vi "FGV Actor Classes-Messages.vi"(8 "Error In":errorcluster, 9 "CS++Messages":refnum<class "Message.lvclass">[](array[class]), 10 "Class Name":string, 11 "Action (read)":T1=enum."read") -> (0 "Error Out":errorcluster, 1 "CS++Messages":refnum<class "Message.lvclass">[](array[class]), 2 "Success":bool, 4 "Class Names":string[](array[string]), 6 "CS++Messages":refnum<class "Message.lvclass">[][](array[class]))   [LabVIEW 2016, in "CS++Base.lvlib"]
doc: "This is a FGV to be used to maintain a list of actor classes and corresponding messages."
uses:
  CS++Base.lvlib
  FGV Action.ctl
  <vilib>/ActorFramework/Message/Message.lvclass
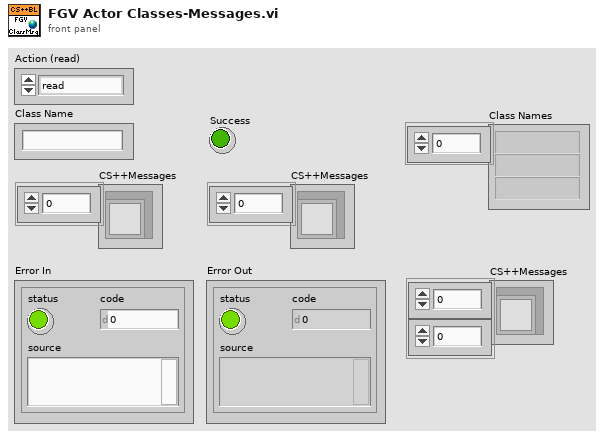
[diagram p1: front panel]
types:
  T1 = typedef "CS++Base.lvlib/FGV Action.ctl" = enum16{"add", "replace", "read", "remove", "reset", "get attributes"}
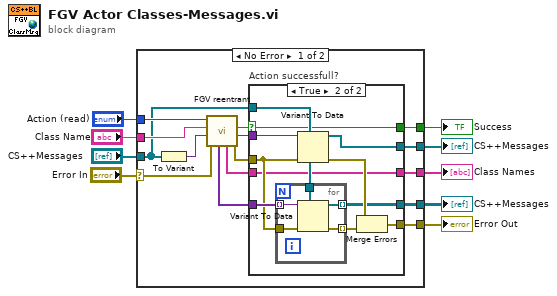
[diagram p0: block diagram]
diagram:
  n1 = case shown="No Error" "Error In" {
    selector: "Error In" -> [w23 w43]
    tunnel: "Action (read)" -> [w24 _]
    tunnel: "Class Name" -> [w22 _]
    tunnel: "CS++Messages" -> [w19 w44]
    tunnel: [w16 w43] -> w5
    tunnel: [w15 _] -> w4
    tunnel: [w14 _] -> w3
    tunnel: [w11 _] -> w2
    tunnel: [w10 w44] -> w1
    frame No Error {
      n2 = To Variant(anything=w19) -> (Variant=w21:variant)
      n3 = call "FGV reentrant.vi"("Error In"=w23, "Data in"=w21, "Attribute Name"=w22, "Action (read)"=w24) -> ("Error Out"=w17:errorcluster, "Data out"=w20:variant, "Success"=w12:bool, "Attribute Names"=w13:string[], "Attribute Values"=w18:variant[])  [unwired: 3 in]
      n4 = case "Action successfull?" shown="True" w12 {
        selector: w12 -> [w26 w28]
        tunnel: w20 -> [_ w37]
        tunnel: w19 -> [_ w36]
        tunnel: w18 -> [_ w35]
        tunnel: w17 -> [w25 w34]
        tunnel: [w25 w31] -> w16
        tunnel: [_ w30] -> w15
        tunnel: [_ w29] -> w14
        tunnel: w13 -> [_ w29]
        tunnel: [w26 w28] -> w11
        tunnel: [_ w27] -> w10
        frame False {
        }
        frame True {
          n5 = for {
            tunnel: w36 -> [w42]
            tunnel: w35 -> [w41] mode=indexing
            tunnel: w34 -> [w40]
            tunnel: [w39] -> w33 mode=indexing
            tunnel: [w38] -> w30 mode=indexing
            n6 = Variant To Data(error in=w40, type=w42, Variant=w41) -> (data=w38:refnum<class "Message.lvclass">[], error out=w39:errorcluster)
          }
          n7 = Variant To Data(error in=w34, type=w36, Variant=w37) -> (data=w27:refnum<class "Message.lvclass">[], error out=w32:errorcluster)
          n8 = Merge Errors(w32, w33) -> (w31:errorcluster)
        }
      }
    }
    frame Error {
    }
  }
  "Error Out" <- w5
  "Class Names" <- w3
  "CS++Messages" <- w4
  "Success" <- w2
  "CS++Messages" <- w1
